vi "LogEnable.vi"(8 "error in (no error)":errorcluster, 10 "Log?":bool, 11 "GUI Actor in":refnum<class "GUI Actor.lvclass">) -> (0 "error out":errorcluster, 3 "GUI Actor out":refnum<class "GUI Actor.lvclass">)   [LabVIEW 2019, in "GUI Actor.lvlib" / "GUI Actor.lvclass"]
uses:
  GUI Actor.lvclass
  GUI Actor.lvclass/GUI Actor.ctl
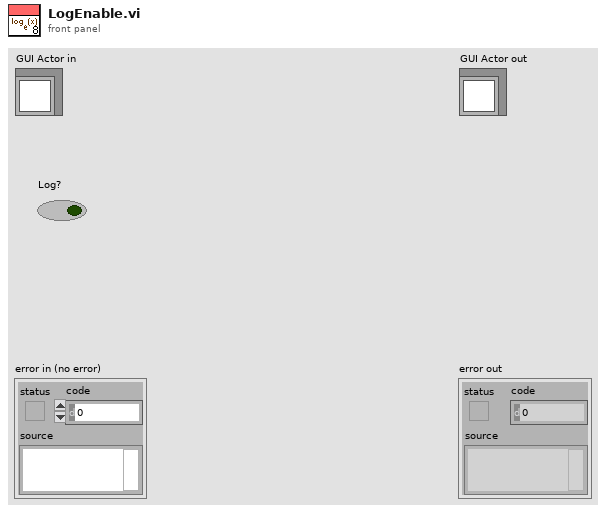
[diagram p1: front panel]
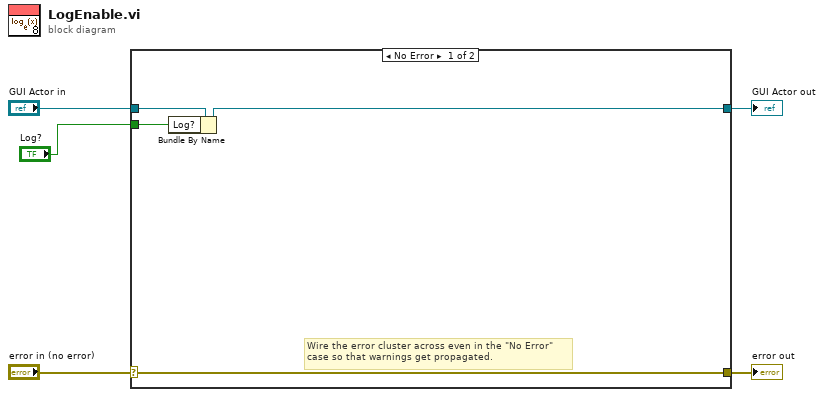
[diagram p0: block diagram]
diagram:
  n1 = case shown="No Error" "error in (no error)" {
    selector: "error in (no error)" -> [w8 w11]
    tunnel: [w8 w11] -> w4
    tunnel: [w7 w10] -> w2
    tunnel: "GUI Actor in" -> [w9 w10]
    tunnel: "Log?" -> [w6 _]
    frame No Error {
      # "Wire the error cluster across even in the \"No Error\"\ncase so that warnings get propagated."
      n2 = Bundle By Name(cluster=w9, "Log?"=w6) -> (w7:refnum<class "GUI Actor.lvclass">)
    }
    frame Error {
    }
  }
  "error out" <- w4
  "GUI Actor out" <- w2
